vi "Serialize - JSON.vi"(8 "error in":errorcluster, 11 "CRDS Cell Data in":refnum<class "CRDS Cell Data.lvclass">) -> (0 "error out":errorcluster, 2 "Serialized JSON":string, 3 "CRDS Cell Data out":refnum<class "CRDS Cell Data.lvclass">)   [LabVIEW 2016, in "CRDS Lib.lvlib" / "CRDS Cell Data.lvclass"]
uses:
  CRDS Cell Data.lvclass
  Cell/extParam Ctl.ctl
  Cell/hkParam Ctl.ctl
  CRDS Cell Data.lvclass/CRDS Cell Data.ctl
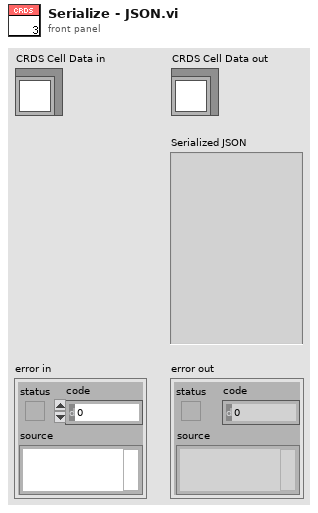
[diagram p1: front panel]
types:
  T1 = typedef "CRDS Lib.lvlib/CRDS Cell Data.lvclass/extParam Ctl.ctl" = cluster{"Tau":sgl, "Tau0cor":sgl, "ext":sgl, "extCorr":sgl, "stdevTau":sgl, "eTau":sgl, "taucorr":sgl, "Tau0":sgl, "max":sgl}
  T2 = typedef "CRDS Lib.lvlib/CRDS Cell Data.lvclass/hkParam Ctl.ctl" = cluster{"rhDilFac":sgl, "Q":sgl, "Tmean":sgl, "extDilFac":sgl, "rhCell":sgl, "P":sgl, "T":sgl}
  T3 = cluster{"extParam":T1, "hkData":T2, "Ringdowns":i16[][]}
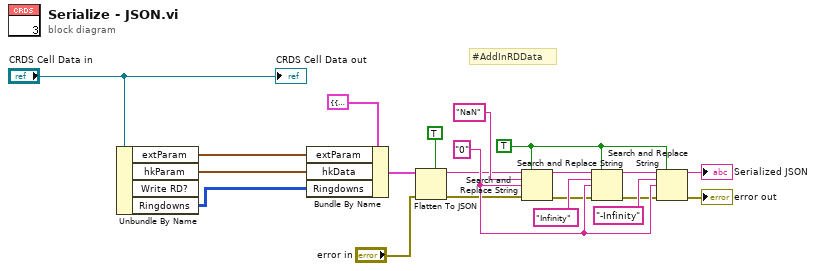
[diagram p0: block diagram]
diagram:
  w10 = "0" ("replace string (\"\")")
  w8 = TRUE ("replace all? (F)")
  # "#AddInRDData"
  n1 = Unbundle By Name("CRDS Cell Data in") -> ("extParam"=w19:T1, "hkParam"=w18:T2, "Ringdowns"=w15:i16[][])  [unwired: 1 out]
  n2 = Bundle By Name(cluster=T3 {"extParam"={"Tau"=0.0, "Tau0cor"=0.0, "ext"=0.0, "extCorr"=0.0, "stdevTau"=0.0, "eTau"=0.0, "taucorr"=0.0, "Tau0"=0.0, "max"=0.0}, "hkData"={"rhDilFac"=0.0, "Q"=0.0, "Tmean"=0.0, "extDilFac"=0.0, "rhCell"=0.0, "P"=0.0, "T"=0.0}, "Ringdowns"=[]} ("CellData"), "extParam"=w19, "hkData"=w18, "Ringdowns"=w15) -> (w17:T3)
  n3 = Flatten To JSON(enable LabVIEW extensions? (T)=TRUE, anything=w17, error in (no error)="error in") -> (JSON string=w4:string, 11:w3:errorcluster)
  n4 = Search and Replace String(replace all?=w8, input string=w4, search string="NaN", replace string=w10, error in=w3) -> (result string=w12:string, error out=w6:errorcluster)  [unwired: 3 in, 2 out]
  n5 = Search and Replace String(replace all?=w8, input string=w12, search string="Infinity", replace string=w10, error in=w6) -> (result string=w11:string, error out=w5:errorcluster)  [unwired: 3 in, 2 out]
  n6 = Search and Replace String(replace all?=w8, input string=w11, search string="-Infinity", replace string=w10, error in=w5) -> (result string=→"Serialized JSON":string, error out=→"error out":errorcluster)  [unwired: 3 in, 2 out]
  "CRDS Cell Data out" <- "CRDS Cell Data in"
